vi "Telnet_RW_wResp_v2.vi"(5 "report_path":path, 6 "bytes to read (1024)":i32=1024, 8 "error in (no error)":errorcluster, 9 "expected string":string, 10 "Command":string) -> (0 "error out":errorcluster, 1 "String found?":bool, 2 "string out":string, 3 "connection ID out":refnum<k5>)   [LabVIEW 2018]
doc: "This VI sends a command using telnet and verifies the response is the expected one."
panel:
  out "offset":i32
  in  "command end":string="->"
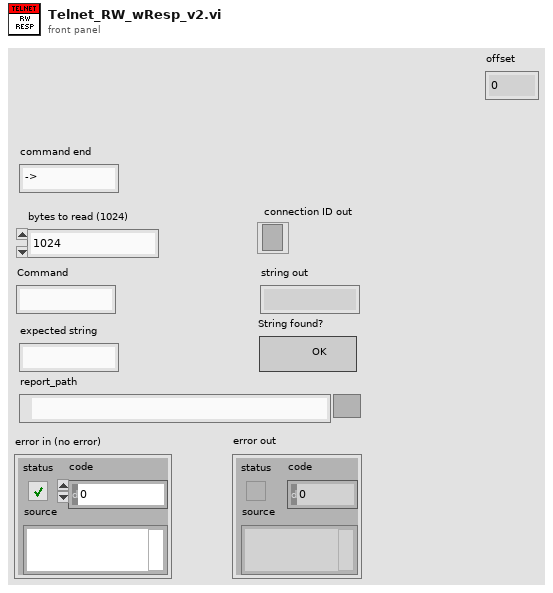
[diagram p1: front panel]
types:
  T1 = enum16{"Standard", "Buffered", "CRLF", "Immediate"}
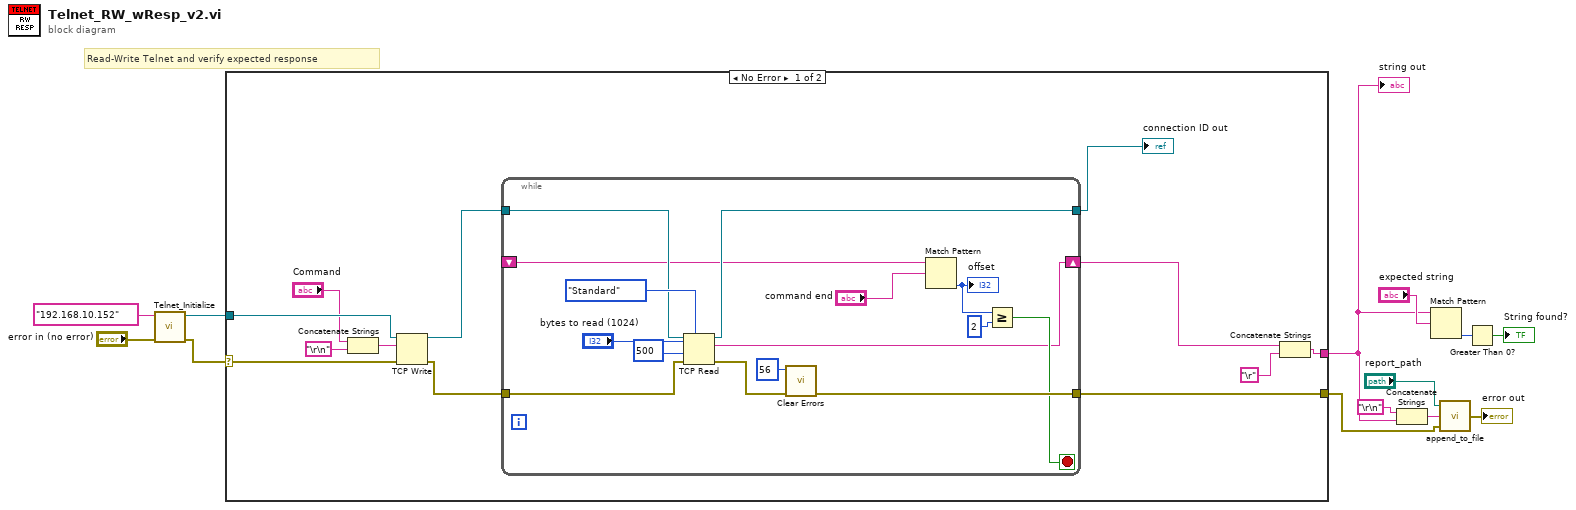
[diagram p0: block diagram]
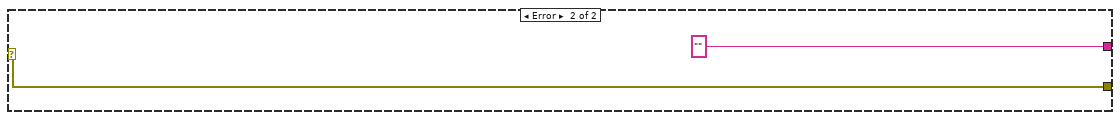
[diagram p2: hidden frame]
diagram:
  # "Read-Write Telnet and verify expected response"
  n1 = call "Telnet_Initialize.vi"("error in (no error)"="error in (no error)", "Address"="192.168.10.152") -> ("error out"=w2:errorcluster, "connection ID out"=w1:refnum<k5>)  [unwired: 8 in]
  n2 = case shown="No Error" w2 {
    selector: w2 -> [w16 w41]
    tunnel: [w23 ""] -> w6
    tunnel: [w22 w41] -> w5
    tunnel: w1 -> [w17 _]
    frame No Error {
      n3 = Concatenate Strings("Command", "\r\n") -> (w21:string)
      n4 = TCP Write(connection ID=w17, data in=w21, error in (no error)=w16) -> (connection ID out=w19:refnum<k5>, error out=w18:errorcluster)  [unwired: 1 in, 1 out]
      n5 = while {
        shift-right: [w27] -> w14
        shift-left: _ -> [w26]
        tunnel: w19 -> [w32]
        tunnel: [w35] -> w25
        tunnel: w18 -> [w34]
        tunnel: [w33] -> w22
        stop <- w28 stop-if-true
        n6 = TCP Read(connection ID=w32, bytes to read="bytes to read (1024)", error in (no error)=w34, 7:T1."Standard" ("mode (standard)"), 9:500 ("timeout ms (25000)")) -> (connection ID out=w35:refnum<k5>, data out=w27:string, error out=w37:errorcluster)
        n7 = call "Clear Errors.vi"("error in (no error)"=w37, "specific error code to clear (0: all)"=56) -> ("error out"=w33:errorcluster)  [unwired: 4 in, 1 out]
        n8 = Match Pattern(string=w26, regular expression="command end") -> (offset past match=w30:i32)  [unwired: 1 in, 3 out]
        "offset" <- w30
        n9 = Greater Or Equal?(x=w30, y=2) -> (x >= y?=w28:bool)
      }
      "connection ID out" <- w25
      n10 = Concatenate Strings(w14, "\r") -> (w23:string)
    }
    frame Error {
    }
  }
  "string out" <- w6
  n11 = Concatenate Strings("\r\n", w6) -> (w11:string)
  n12 = Match Pattern(string=w6, regular expression="expected string") -> (offset past match=w9:i32)  [unwired: 1 in, 3 out]
  n13 = call "append_to_file.vi"("error in (no error)"=w5, "text"=w11, "file_path"="report_path") -> ("error out"=→"error out":errorcluster)
  n14 = Greater Than 0?(x=w9) -> (x > 0?=→"String found?":bool)
